vi "Report Previous Error.vi"(8 "error in (no error)":errorcluster, 11 "Module in":refnum<class "Module.lvclass">) -> (0 "error out":errorcluster, 3 "Module out":refnum<class "Module.lvclass">)   [LabVIEW 2020, in "Volatus.lvlib" / "Module.lvclass"]
uses:
  Module.lvclass
  Module.lvclass/Module.ctl
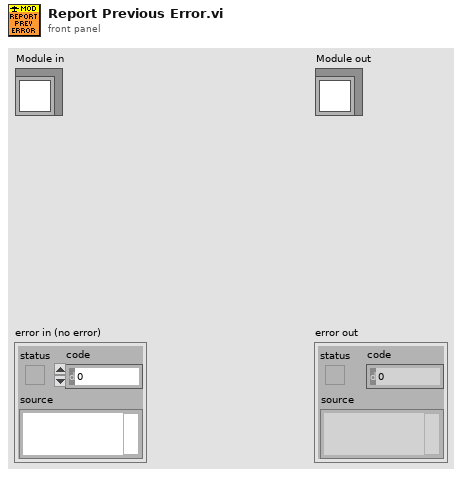
[diagram p1: front panel]
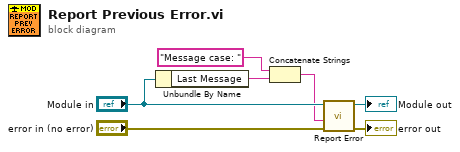
[diagram p0: block diagram]
diagram:
  n1 = Unbundle By Name("Module in") -> ("Last Message"=w6:string)
  n2 = Concatenate Strings("Message case: " ("string"), w6) -> (w3:string)
  n3 = call "Report Error.vi"("error in (no error)"="error in (no error)", "Message (None)"=w3, "Module in"="Module in") -> ("error out"=→"error out":errorcluster, "Module out"=→"Module out":refnum<class "Module.lvclass">)  [unwired: 7 in]
